vi "share data state machine.vi"(6 "Share data command":T7=enum."Write data", 8 "error in (no error)":errorcluster, 10 "Selected Shared Data":T3, 11 "Write data cluster in":T4) -> (0 "error out":errorcluster, 1 "Data from shared sources":T1 {"Sensor array"."scaled" format="%.2f"; "Sensor array"."voltage" format="%.4f"; "Time" format="%<%I:%M:%S%2u %p\n%m/%d/%Y>T"}, 2 "Available shared data":T5 {"Shared Data"."scaled" format="%.2f"}, 3 "My Data":T6 {"scaled" format="%.2f"}, 4 "Shared data names (unit)":string[](array[string]), 5 "read error":bool, 7 "Write data cluster out":T4)   [LabVIEW 2015]
uses:
  share data command.ctl
  shared data (name value unit).ctl
  write data cluster.ctl
  available share data.ctl
  selected shared data.ctl
  TCP DAQ/Sensor data.ctl
  DAQ configuration/sensor cluster.ctl
  Process Controller 3.0/Calibration and Function folders.ctl
  buffer.ctl
  <vilib>/Utility/config.llb/Read Key (Double).vi
  <vilib>/Utility/config.llb/Read Key (Path).vi
  <vilib>/Utility/config.llb/Read Key (U32).vi
  <vilib>/Utility/config.llb/Read Key (String).vi
  <vilib>/Utility/config.llb/Write Key (Double).vi
  <vilib>/Utility/config.llb/Write Key (Path).vi
  <vilib>/Utility/config.llb/Write Key (U32).vi
  <vilib>/Utility/config.llb/Write Key (String).vi
  <vilib>/Utility/config.llb/NI_LVConfig.lvlib
panel:
  out "my shared data file path":path
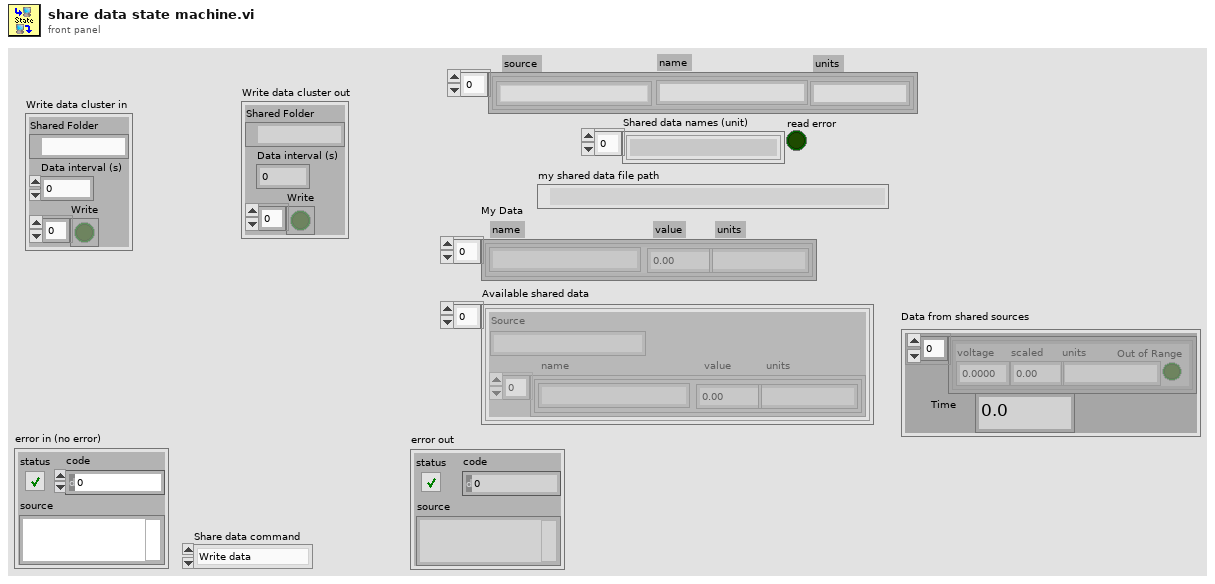
[diagram p1: front panel]
types:
  T1 = typedef "Sensor data.ctl" = cluster{" Sensor array":T2[], "Time":dbl}
  T2 = typedef "sensor cluster.ctl" = cluster{"voltage":sgl, "scaled":sgl, "units":string, "Out of Range":bool}
  T3 = typedef "selected shared data.ctl" = cluster{"Source":string, "name":string, "units":string}[]
  T4 = typedef "write data cluster.ctl" = cluster{"Data interval (s)":sgl, "Shared Folder":path, "Write":bool[]}
  T5 = typedef "available share data.ctl" = cluster{"Source":string, "Shared Data":T6}[]
  T6 = typedef "shared data (name value unit).ctl" = cluster{"name":string, "units":string, "scaled":sgl}[]
  T7 = typedef "share data command.ctl" = enum16{"Initialize from ini", "Update ini", "Write data", "Read data", "List my data", "List shared data", "Close"}
  T8 = typedef "Calibration and Function folders.ctl" = enum16{"Sensors", "Functions", "Config File", "PublicAppFolder", "New ini File", "Set Config File", "Delete ini File"}
  T9 = typedef "buffer.ctl" = enum16{"write", "read", "read merge"}
  T10 = cluster{"Controls[][0]":refnum<vi>, "Controls[][1]":refnum<vi>, "Controls[][2]":refnum<vi>}
  T11 = typedef "NI_LVConfig.lvlib/Config Data RefNum.ctl" = refnum<k1>
  T12 = cluster{"name":string, "units":string, "scaled":sgl}
  T13 = cluster{"name":string, cluster{"name":string, "units":string, "scaled":sgl}[]}
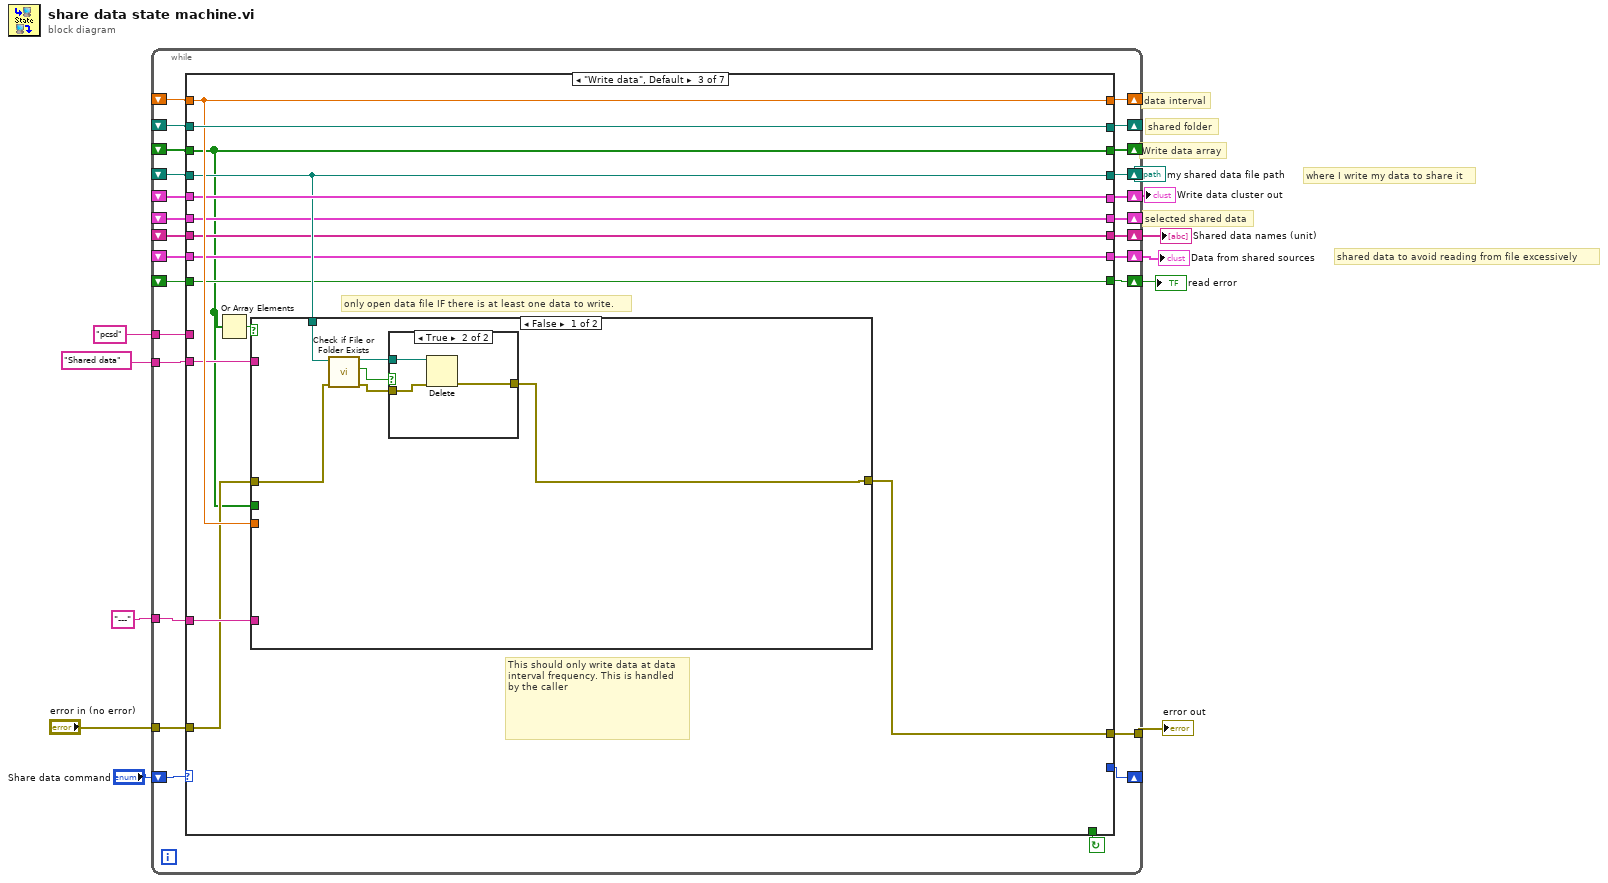
[diagram p0: block diagram]
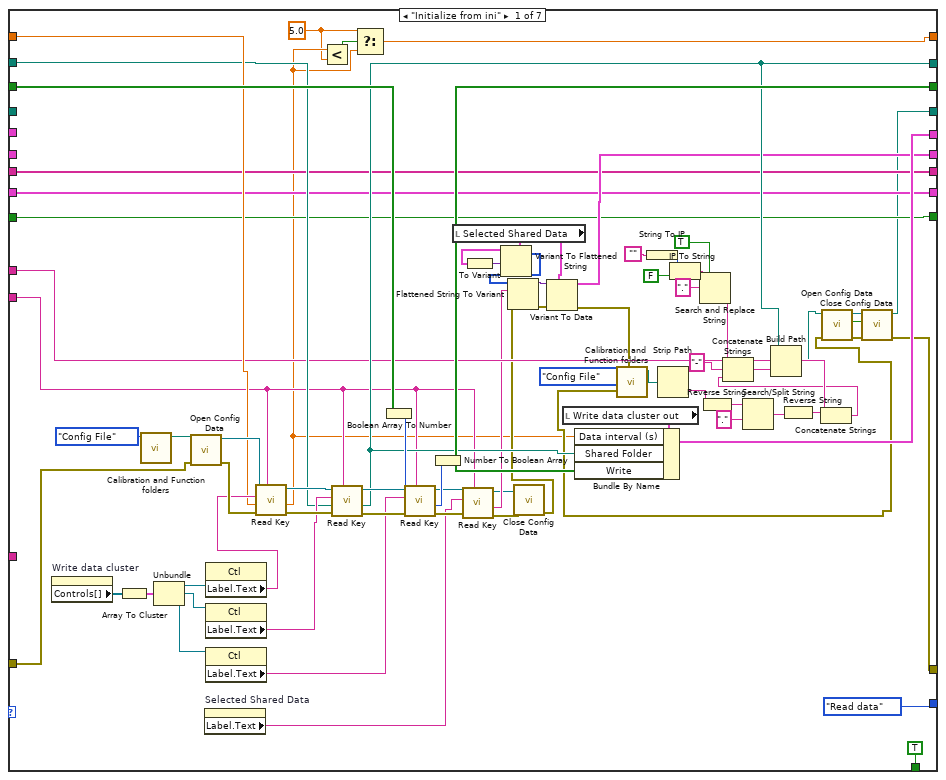
[diagram p2: hidden frame]
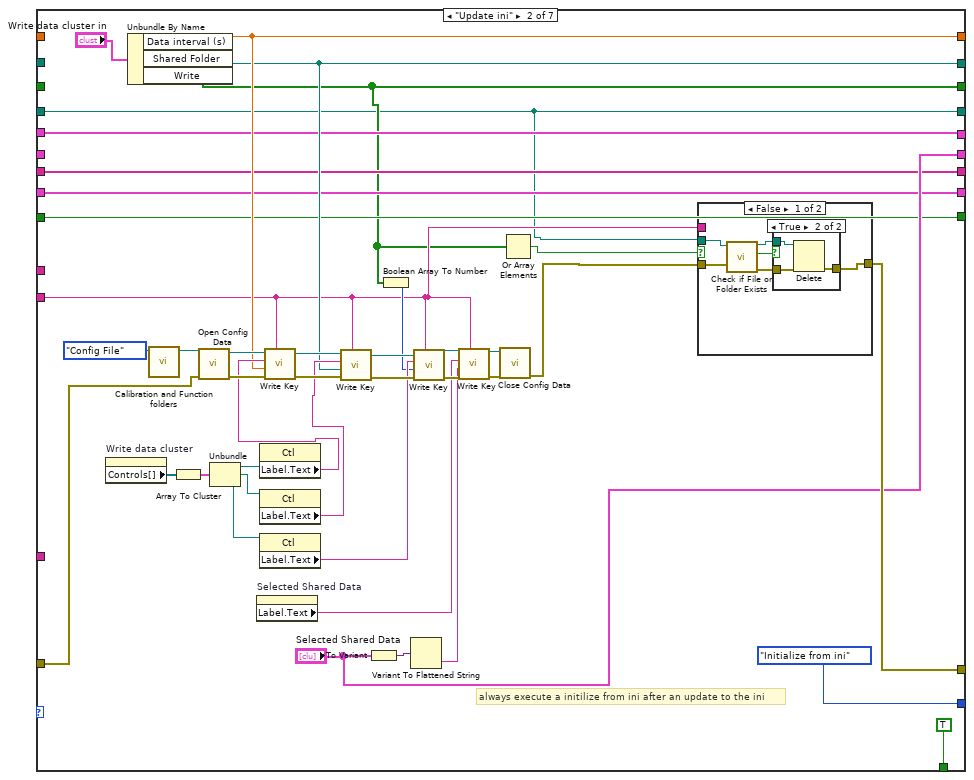
[diagram p3: hidden frame]
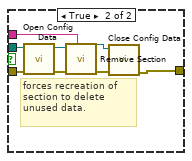
[diagram p5: hidden frame]
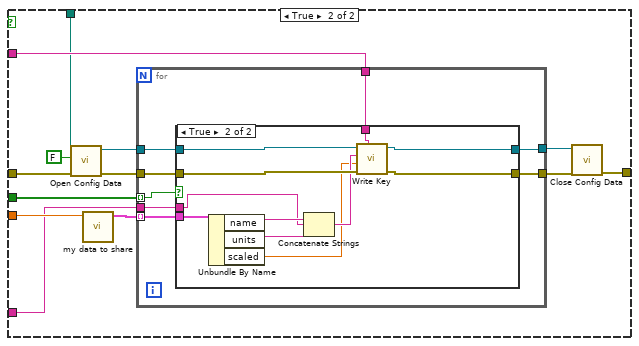
[diagram p7: hidden frame]
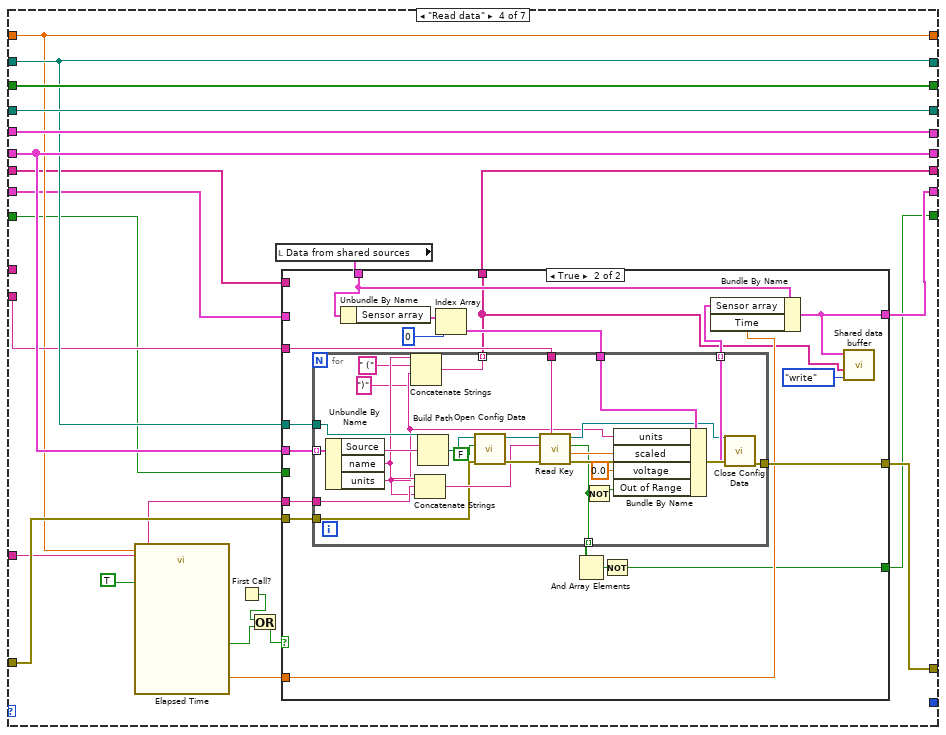
[diagram p9: hidden frame]
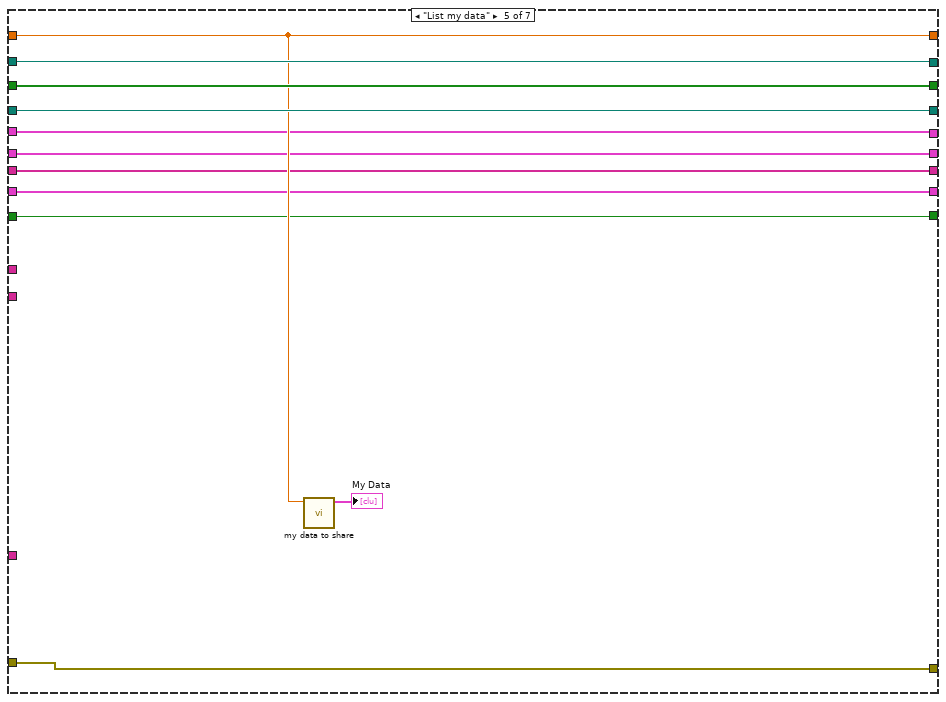
[diagram p11: hidden frame]
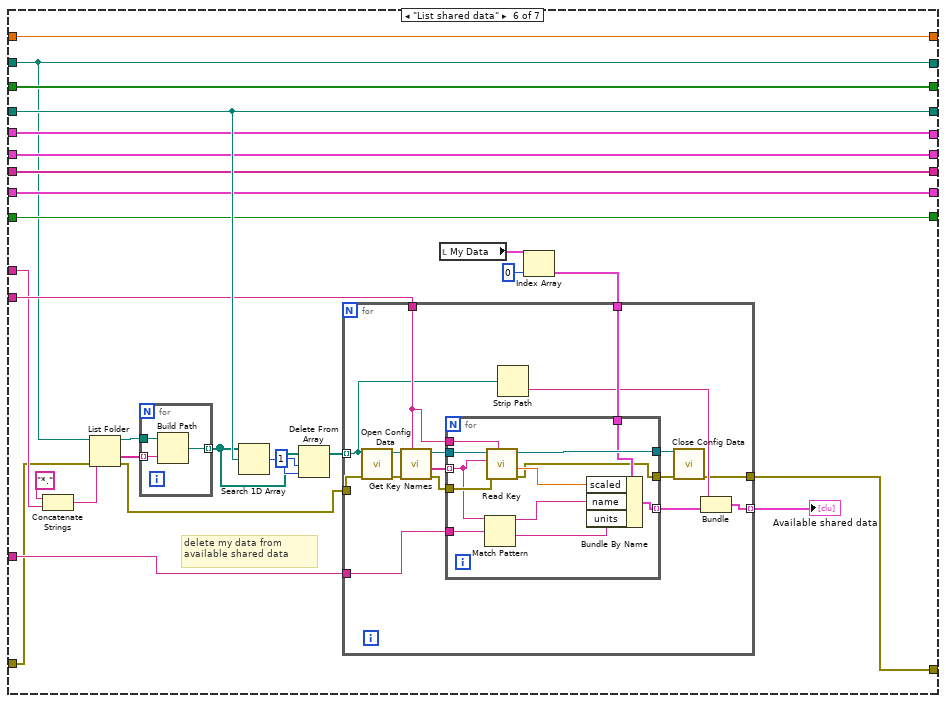
[diagram p12: hidden frame]
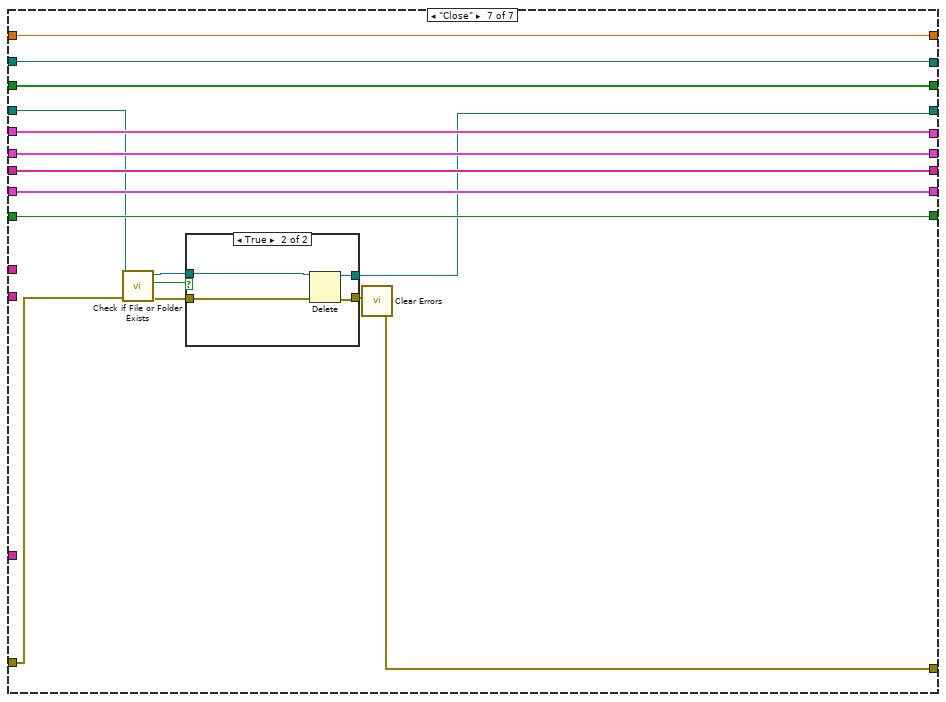
[diagram p13: hidden frame]
diagram:
  # "shared data to avoid reading from file excessively"
  # "selected shared data"
  # "Write data array"
  # "where I write my data to share it"
  # "shared folder"
  # "data interval"
  n1 = while {
    tunnel: [w37] -> w11
    tunnel: "error in (no error)" -> [w36]
    shift-right: [w35] -> _
    shift-left: _ -> [w34]
    shift-right: [w33] -> _
    shift-left: _ -> [w32]
    shift-right: [w31] -> w4
    shift-left: _ -> [w30]
    tunnel: "Shared data" ("section") -> [w29]
    shift-right: [w28] -> _
    shift-left: _ -> [w27]
    shift-right: [w26] -> w8
    shift-left: _ -> [w25]
    tunnel: "pcsd" ("pattern") -> [w24]
    shift-right: [w23] -> _
    shift-left: "Share data command" -> [w21]
    tunnel: "---" ("unit delimiter") -> [w20]
    shift-right: [w19] -> _
    shift-left: _ -> [w18]
    shift-right: [w17] -> w3
    shift-left: _ -> [w15]
    shift-right: [w16] -> w2
    shift-left: _ -> [w14]
    shift-right: [w13] -> w1
    shift-left: _ -> [w12]
    stop <- w22 continue-if-true
    n2 = case shown="\"Write data\", Default" w21 {
      tunnel: [w42 w128 w177 w243 w308 w324 w367] -> w37
      tunnel: w36 -> [w95 w144 w178 w244 w308 w309 w372]
      tunnel: [w40 w133 w183 w241 w303 w335 w382] -> w35
      tunnel: w34 -> [w81 _ w183 w241 w303 w335 w382]
      tunnel: [w79 w132 w184 w246 w307 w315 w381] -> w33
      tunnel: w32 -> [w80 _ w184 w246 w307 w315 w381]
      tunnel: [w44 w112 w179 w250 w306 w333 w368] -> w31
      tunnel: w30 -> [_ w112 w179 w250 w306 w333 w373]
      tunnel: w29 -> [w68 w126 w182 w245 _ w329 _]
      tunnel: [w83 w115 w172 w249 w305 w334 w380] -> w28
      tunnel: w27 -> [w87 _ w172 w249 w305 w334 w380]
      tunnel: [w78 w131 w181 w248 w302 w323 w379] -> w26
      tunnel: w25 -> [_ w131 w181 w248 w302 w323 w379]
      tunnel: w24 -> [w74 _ _ _ _ w321 _]
      tunnel: [share_data_command."Read data" ("Share data command") share_data_command."Initialize from ini" ("Share data command") _ _ _ _ _] -> w23
      tunnel: [TRUE TRUE _ _ _ _ _] -> w22
      tunnel: w20 -> [_ _ w180 w242 _ w320 _]
      tunnel: [w64 "Selected Shared Data" w176 w247 w301 w319 w377] -> w19
      tunnel: w18 -> [_ _ w176 w247 w301 w319 w377]
      tunnel: [w56 w119 w175 w239 w300 w318 w376] -> w17
      tunnel: [w55 w118 w174 w234 w299 w317 w375] -> w16
      tunnel: w15 -> [w56 w119 w175 w238 w300 w318 w376]
      tunnel: w14 -> [w55 w118 w174 w237 w299 w317 w375]
      tunnel: [w54 w117 w173 w233 w298 w316 w374] -> w13
      tunnel: w12 -> [w54 w117 w173 w232 w298 w316 w374]
      frame "Initialize from ini" {
        w38 = 5.0 ("t")
        n3 = property on="Write data cluster" class="Clust (strict)"() -> ("Controls[]"=w94:refnum<vi>[])  [unwired: 2 in, 2 out]
        n4 = Array To Cluster(array=w94) -> (cluster=w93:T10)
        n5 = call "Calibration and Function folders.vi"("Folder"=Calibration_and_Function_folders."Config File") -> ("Selected Folder"=w101:path)  [unwired: 9 in, 1 out]
        n6 = Unbundle(w93) -> ("Controls[][0]"=w92:refnum<vi>, "Controls[][1]"=w91:refnum<vi>, "Controls[][2]"=w90:refnum<vi>)
        n7 = call <vilib>:"Open Config Data.vi"("error in (no error)"=w95, "configuration file path"=w101) -> ("error out"=w102:errorcluster, "refnum"=w103:T11)  [unwired: 7 in, 1 out]
        n8 = property on="Selected Shared Data" class="Arr (strict)"() -> ("Label.Text"=w67:string)  [unwired: 2 in, 2 out]
        n9 = property class="Ctl"(reference=w92) -> ("Label.Text"=w89:string)  [unwired: 1 in, 2 out]
        n10 = property class="Ctl"(reference=w91) -> ("Label.Text"=w88:string)  [unwired: 1 in, 2 out]
        n11 = property class="Ctl"(reference=w90) -> ("Label.Text"=w85:string)  [unwired: 1 in, 2 out]
        n12 = call-poly <vilib>:"Read Key.vi"("section"=w68, "error in (no error)"=w102, "default value"=w81, "key"=w89, "refnum"=w103) -> ("error out"=w97:errorcluster, "value"=w39:dbl, "refnum out"=w99:T11)  [unwired: 3 in, 1 out]
        n13 = Less?(x=w39, y=w38) -> (x < y?=w41:bool)
        n14 = call-poly <vilib>:"Read Key.vi"("section"=w68, "error in (no error)"=w97, "default value"=w80, "key"=w88, "refnum"=w99) -> ("error out"=w96:errorcluster, "value"=w79:path, "refnum out"=w98:T11)  [unwired: 3 in, 1 out]
        n15 = Select(t=w38, s=w41, f=w39) -> (s? t:f=w40:dbl)
        n16 = Boolean Array To Number(Boolean array=w87) -> (number=w84:u32)
        n17 = call-poly <vilib>:"Read Key.vi"("section"=w68, "error in (no error)"=w96, "default value"=w84, "key"=w85, "refnum"=w98) -> ("error out"=w70:errorcluster, "value"=w86:u32, "refnum out"=w62:T11)  [unwired: 3 in, 1 out]
        n18 = Number To Boolean Array(number=w86) -> (Boolean array=w83:bool[])
        n19 = local read "Selected Shared Data"() -> (w57:T3)
        n20 = call-poly <vilib>:"Read Key.vi"("section"=w68, "error in (no error)"=w70, "key"=w67, "refnum"=w62) -> ("error out"=w69:errorcluster, "value"=w66:string, "refnum out"=w63:T11)  [unwired: 4 in, 1 out]
        n21 = To Variant(anything=w57) -> (Variant=w61:variant)
        n22 = Variant To Flattened String(Variant=w61) -> (1:w60:i16[])  [unwired: 1 out]
        n23 = call <vilib>:"Close Config Data.vi"("error in (no error)"=w69, "refnum"=w63) -> ("error out"=w59:errorcluster)  [unwired: 8 in, 1 out]
        n24 = Flattened String To Variant(4:w59, 6:w66, 7:w60) -> (0:w58:errorcluster, 3:w65:variant)
        n25 = Variant To Data(error in=w58, type=w57, Variant=w65) -> (data=w64:T3, error out=w43:errorcluster)
        n26 = local read "Write data cluster out"() -> (w82:T4)
        n27 = Bundle By Name(cluster=w82, "Data interval (s)"=w39, "Shared Folder"=w79, "Write"=w83) -> (w78:T4)
        n28 = call "Calibration and Function folders.vi"("Folder"=Calibration_and_Function_folders."Config File") -> ("Selected Folder"=w107:path)  [unwired: 9 in, 1 out]
        n29 = String To IP(1:"") -> (0:w111:u32)
        n30 = Strip Path(path=w107) -> (name=w75:string)  [unwired: 1 out]
        n31 = IP To String(1:FALSE ("dot notation? (F)"), 2:w111) -> (0:w105:string)
        n32 = Search and Replace String(replace all?=TRUE ("replace all? (F)"), input string=w105, search string=".") -> (result string=w51:string)  [unwired: 5 in, 3 out]
        n33 = Reverse String(1:w75) -> (0:w77:string)
        n34 = Search/Split String(string=w77, search string/char (-)=".") -> (match + rest of string=w71:string)  [unwired: 1 in, 2 out]
        n35 = Reverse String(1:w71) -> (0:w73:string)
        n36 = Concatenate Strings(w73, w74) -> (w72:string)
        n37 = Concatenate Strings(w51, "-" ("string"), w72) -> (w106:string)
        n38 = Build Path(base path=w79, name or relative path=w106) -> (appended path=w45:path)
        n39 = call <vilib>:"Open Config Data.vi"("error in (no error)"=w43, "configuration file path"=w45) -> ("error out"=w46:errorcluster, "file created?"=w47:bool, "refnum"=w48:T11)  [unwired: 7 in]
        n40 = call <vilib>:"Close Config Data.vi"("error in (no error)"=w46, "write file if changed (T)"=w47, "refnum"=w48) -> ("error out"=w42:errorcluster, "file path"=w44:path)  [unwired: 7 in]
      }
      frame "Update ini" {
        # "always execute a initilize from ini after an update to the ini"
        n41 = property on="Write data cluster" class="Clust (strict)"() -> ("Controls[]"=w142:refnum<vi>[])  [unwired: 2 in, 2 out]
        n42 = Unbundle By Name("Write data cluster in") -> ("Data interval (s)"=w133:sgl, "Shared Folder"=w132:path, "Write"=w115:bool[])
        n43 = call "Calibration and Function folders.vi"("Folder"=Calibration_and_Function_folders."Config File") -> ("Selected Folder"=w150:path)  [unwired: 9 in, 1 out]
        n44 = Array To Cluster(array=w142) -> (cluster=w141:T10)
        n45 = call <vilib>:"Open Config Data.vi"("error in (no error)"=w144, "configuration file path"=w150) -> ("error out"=w151:errorcluster, "refnum"=w152:T11)  [unwired: 7 in, 1 out]
        n46 = Unbundle(w141) -> ("Controls[][0]"=w140:refnum<vi>, "Controls[][1]"=w139:refnum<vi>, "Controls[][2]"=w138:refnum<vi>)
        n47 = property on="Selected Shared Data" class="Arr (strict)"() -> ("Label.Text"=w123:string)  [unwired: 2 in, 2 out]
        n48 = property class="Ctl"(reference=w140) -> ("Label.Text"=w137:string)  [unwired: 1 in, 2 out]
        n49 = property class="Ctl"(reference=w139) -> ("Label.Text"=w136:string)  [unwired: 1 in, 2 out]
        n50 = property class="Ctl"(reference=w138) -> ("Label.Text"=w135:string)  [unwired: 1 in, 2 out]
        n51 = call-poly <vilib>:"Write Key.vi"("section"=w126, "error in (no error)"=w151, "value"=w133, "key"=w137, "refnum"=w152) -> ("error out"=w146:errorcluster, "refnum out"=w148:T11)  [unwired: 4 in, 1 out]
        n52 = call-poly <vilib>:"Write Key.vi"("section"=w126, "error in (no error)"=w146, "value"=w132, "key"=w136, "refnum"=w148) -> ("error out"=w145:errorcluster, "refnum out"=w147:T11)  [unwired: 4 in, 1 out]
        n53 = To Variant(anything="Selected Shared Data") -> (Variant=w122:variant)
        n54 = Boolean Array To Number(Boolean array=w115) -> (number=w134:u32)
        n55 = Variant To Flattened String(Variant=w122) -> (data string=w121:string)  [unwired: 1 out]
        n56 = call-poly <vilib>:"Write Key.vi"("section"=w126, "error in (no error)"=w145, "value"=w134, "key"=w135, "refnum"=w147) -> ("error out"=w125:errorcluster, "refnum out"=w127:T11)  [unwired: 4 in, 1 out]
        n57 = call-poly <vilib>:"Write Key.vi"("section"=w126, "error in (no error)"=w125, "value"=w121, "key"=w123, "refnum"=w127) -> ("error out"=w124:errorcluster, "refnum out"=w114:T11)  [unwired: 4 in, 1 out]
        n58 = call <vilib>:"Close Config Data.vi"("error in (no error)"=w124, "refnum"=w114) -> ("error out"=w113:errorcluster)  [unwired: 8 in, 1 out]
        n59 = Or Array Elements(Boolean array=w115) -> (logical OR=w116:bool)
        n60 = case shown="False" w116 {
          tunnel: [w158 w168] -> w128
          tunnel: w112 -> [w157 w167]
          tunnel: w113 -> [w156 w166]
          tunnel: w126 -> [_ w163]
          frame False {
            n61 = call <vilib>:"Check if File or Folder Exists.vi"("error in (no error)"=w156, "path"=w157) -> ("error out"=w154:errorcluster, "file or folder exists?"=w155:bool, "dup path"=w153:path)  [unwired: 7 in]
            n62 = case shown="True" w155 {
              tunnel: [w159 w162] -> w158
              tunnel: w154 -> [w159 w161]
              tunnel: w153 -> [_ w160]
              frame False {
              }
              frame True {
                n63 = Delete(path (use dialog)=w160, error in=w161) -> (error out=w162:errorcluster)  [unwired: 3 in, 2 out]
              }
            }
          }
          frame True {
            # "forces recreation of section to delete unused data."
            n64 = call <vilib>:"Open Config Data.vi"("error in (no error)"=w166, "configuration file path"=w167) -> ("error out"=w164:errorcluster, "refnum"=w165:T11)  [unwired: 7 in, 1 out]
            n65 = call <vilib>:"Remove Section.vi"("section"=w163, "error in (no error)"=w164, "refnum"=w165) -> ("error out"=w169:errorcluster, "refnum out"=w170:T11)  [unwired: 6 in, 1 out]
            n66 = call <vilib>:"Close Config Data.vi"("error in (no error)"=w169, "refnum"=w170) -> ("error out"=w168:errorcluster)  [unwired: 8 in, 1 out]
          }
        }
      }
      frame "Write data", Default {
        # "only open data file IF there is at least one data to write."
        # "This should only write data at data interval frequency. This is handled by the caller"
        n67 = Or Array Elements(Boolean array=w172) -> (logical OR=w171:bool)
        n68 = case shown="False" w171 {
          tunnel: w183 -> [_ w207]
          tunnel: w182 -> [_ w205]
          tunnel: w172 -> [_ w204]
          tunnel: w180 -> [_ w203]
          tunnel: w179 -> [w190 w202]
          tunnel: w178 -> [w185 w201]
          tunnel: [w186 w196] -> w177
          frame False {
            n69 = call <vilib>:"Check if File or Folder Exists.vi"("error in (no error)"=w185, "path"=w190) -> ("error out"=w187:errorcluster, "file or folder exists?"=w189:bool, "dup path"=w188:path)  [unwired: 7 in]
            n70 = case shown="True" w189 {
              tunnel: w188 -> [_ w194]
              tunnel: w187 -> [w191 w193]
              tunnel: [w191 w192] -> w186
              frame False {
              }
              frame True {
                n71 = Delete(path (use dialog)=w194, error in=w193) -> (error out=w192:errorcluster)  [unwired: 3 in, 2 out]
              }
            }
          }
          frame True {
            n72 = call <vilib>:"Open Config Data.vi"("error in (no error)"=w201, "create file if necessary (T)"=FALSE, "configuration file path"=w202) -> ("error out"=w200:errorcluster, "refnum"=w199:T11)  [unwired: 6 in, 1 out]
            n73 = call "my data to share.vi"("Data interval (s)"=w207) -> ("Shared Data"=w206:T6)  [unwired: 10 in]
            n74 = for {
              tunnel: [w215] -> w198
              tunnel: w199 -> [w214]
              tunnel: w200 -> [w213]
              tunnel: [w212] -> w197
              tunnel: w206 -> [w209] mode=indexing
              tunnel: w205 -> [w211]
              tunnel: w204 -> [w210] mode=indexing
              tunnel: w203 -> [w208]
              n75 = case shown="True" w210 {
                tunnel: [w217 w228] -> w215
                tunnel: w214 -> [w217 w227]
                tunnel: w213 -> [w216 w226]
                tunnel: [w216 w225] -> w212
                tunnel: w211 -> [_ w224]
                tunnel: w209 -> [_ w223]
                tunnel: w208 -> [_ w218]
                frame False {
                }
                frame True {
                  n76 = Unbundle By Name(w223) -> ("name"=w222:string, "units"=w221:string, "scaled"=w219:sgl)
                  n77 = Concatenate Strings(w222, w218, w221) -> (w220:string)
                  n78 = call-poly <vilib>:"Write Key.vi"("section"=w224, "error in (no error)"=w226, "value"=w219, "key"=w220, "refnum"=w227) -> ("error out"=w225:errorcluster, "refnum out"=w228:T11)  [unwired: 4 in, 1 out]
                }
              }
            }
            n79 = call <vilib>:"Close Config Data.vi"("error in (no error)"=w197, "refnum"=w198) -> ("error out"=w196:errorcluster)  [unwired: 8 in, 1 out]
          }
        }
      }
      frame "Read data" {
        n80 = call "Elapsed Time"("Time Target (s)"=w241, "Auto Reset"=TRUE ("Reset")) -> ("Present (s)"=w236:dbl, "Time has Elapsed"=w230:bool)  [unwired: 10 in, 6 out]
        n81 = First Call?() -> (First Call?: T/F=w231:bool)
        n82 = Or(x=w231, y=w230) -> (x .or. y?=w229:bool)
        n83 = local read "Data from shared sources"() -> (w235:T1)
        n84 = case shown="True" w229 {
          tunnel: w247 -> [_ w272]
          tunnel: w246 -> [_ w271]
          tunnel: w245 -> [_ w270]
          tunnel: w244 -> [w254 w269]
          tunnel: [w254 w268] -> w243
          tunnel: w242 -> [_ w267]
          tunnel: [w253 w255] -> w239
          tunnel: w238 -> [w253 _]
          tunnel: w237 -> [w252 _]
          tunnel: w236 -> [_ w261]
          tunnel: w235 -> [_ w262]
          tunnel: [w252 w260] -> w234
          tunnel: [w251 w256] -> w233
          tunnel: w232 -> [w251 _]
          frame False {
          }
          frame True {
            n85 = Unbundle By Name(w262) -> ("Sensor array"=w266:T2[])
            n86 = Index Array(array=w266, index=0) -> (element=w264:T2)
            n87 = for {
              tunnel: w272 -> [w297] mode=indexing
              tunnel: w271 -> [w285]
              tunnel: w270 -> [w294]
              tunnel: w269 -> [w286]
              tunnel: [w291] -> w268
              tunnel: w264 -> [w290]
              tunnel: w267 -> [w289]
              tunnel: [w284] -> w263 mode=indexing
              tunnel: [w277] -> w255 mode=indexing
              tunnel: [w274] -> w258 mode=indexing
              n88 = Unbundle By Name(w297) -> ("Source"=w296:string, "name"=w281:string, "units"=w279:string)
              n89 = Concatenate Strings(w281, " (" ("string"), w279, ")" ("string")) -> (w277:string)
              n90 = Concatenate Strings(w281, w289, w279) -> (w288:string)
              n91 = Build Path(base path=w285, name or relative path=w296) -> (appended path=w295:path)
              n92 = call <vilib>:"Open Config Data.vi"("error in (no error)"=w286, "create file if necessary (T)"=FALSE, "configuration file path"=w295) -> ("error out"=w293:errorcluster, "refnum"=w283:T11)  [unwired: 6 in, 1 out]
              n93 = call-poly <vilib>:"Read Key.vi"("section"=w294, "error in (no error)"=w293, "key"=w288, "refnum"=w283) -> ("error out"=w292:errorcluster, "value"=w287:dbl, "found?"=w274:bool, "refnum out"=w282:T11)  [unwired: 4 in]
              n94 = Not(x=w274) -> (.not. x?=w273:bool)
              n95 = Bundle By Name(cluster=w290, "units"=w279, "scaled"=w287, "voltage"=sgl 0.0, "Out of Range"=w273) -> (w284:T2)
              n96 = call <vilib>:"Close Config Data.vi"("error in (no error)"=w292, "refnum"=w282) -> ("error out"=w291:errorcluster)  [unwired: 8 in, 1 out]
            }
            n97 = And Array Elements(Boolean array=w258) -> (logical AND=w257:bool)
            n98 = Not(x=w257) -> (.not. x?=w256:bool)
            n99 = Bundle By Name(cluster=w262, "Sensor array"=w263, "Time"=w261) -> (w260:T1)
            n100 = call "Shared data buffer.vi"("command"=buffer."write", "Shared data names (unit) in"=w255, "Data from shared sources in"=w260) -> ()  [unwired: 6 in, 3 out]
          }
        }
      }
      frame "List my data" {
        n101 = call "my data to share.vi"("Data interval (s)"=w303) -> ("Shared Data"=→"My Data":T6)  [unwired: 10 in]
      }
      frame "List shared data" {
        # "delete my data from available shared data"
        n102 = Concatenate Strings("*." ("pattern"), w321) -> (w314:string)
        n103 = List Folder(path=w315, pattern=w314, error in=w309) -> (path out=w313:path, filenames=w312:string[], error out=w310:errorcluster)  [unwired: 1 in, 1 out]
        n104 = for {
          tunnel: w313 -> [w338]
          tunnel: w312 -> [w337] mode=indexing
          tunnel: [w336] -> w311 mode=indexing
          n105 = Build Path(base path=w338, name or relative path=w337) -> (appended path=w336:path)
        }
        n106 = Search 1D Array(1D array=w311, element=w333) -> (index of element=w332:i32)  [unwired: 1 in]
        n107 = Delete From Array(array=w311, length=1, index=w332) -> (array with subset deleted=w330:path[])  [unwired: 1 out]
        n108 = local read "My Data"() -> (w328:T6)
        n109 = Index Array(array=w328, index=0) -> (element=w326:T12)
        n110 = for {
          tunnel: w330 -> [w345] mode=indexing
          tunnel: w329 -> [w351]
          tunnel: w326 -> [w347]
          tunnel: [w343] -> w325 mode=indexing
          tunnel: w310 -> [w342]
          tunnel: [w340] -> w324
          tunnel: w320 -> [w339]
          n111 = call <vilib>:"Open Config Data.vi"("error in (no error)"=w342, "configuration file path"=w345) -> ("error out"=w354:errorcluster, "refnum"=w353:T11)  [unwired: 7 in, 1 out]
          n112 = call <vilib>:"Get Key Names.vi"("section"=w351, "error in (no error)"=w354, "refnum"=w353) -> ("error out"=w349:errorcluster, "key names"=w350:string[], "refnum out"=w352:T11)  [unwired: 5 in, 1 out]
          n113 = for {
            tunnel: w352 -> [w366]
            tunnel: w351 -> [w365]
            tunnel: w350 -> [w358] mode=indexing
            tunnel: w349 -> [w364]
            tunnel: [w363] -> w348
            tunnel: w347 -> [w362]
            tunnel: [w360] -> w346 mode=indexing
            tunnel: [w359] -> w341
            tunnel: w339 -> [w355]
            n114 = Match Pattern(string=w358, regular expression=w355) -> (before substring=w357:string, after substring=w356:string)  [unwired: 1 in, 2 out]
            n115 = call-poly <vilib>:"Read Key.vi"("section"=w365, "error in (no error)"=w364, "key"=w358, "refnum"=w366) -> ("error out"=w359:errorcluster, "value"=w361:dbl, "refnum out"=w363:T11)  [unwired: 4 in, 1 out]
            n116 = Bundle By Name(cluster=w362, "scaled"=w361, "name"=w357, "units"=w356) -> (w360:T12)
          }
          n117 = Strip Path(path=w345) -> (name=w344:string)  [unwired: 1 out]
          n118 = call <vilib>:"Close Config Data.vi"("error in (no error)"=w341, "refnum"=w348) -> ("error out"=w340:errorcluster)  [unwired: 8 in, 1 out]
          n119 = Bundle("name"=w344, w346) -> (w343:T13)  [unwired: 1 in]
        }
        "Available shared data" <- w325
      }
      frame "Close" {
        n120 = call <vilib>:"Check if File or Folder Exists.vi"("error in (no error)"=w372, "path"=w373) -> ("error out"=w369:errorcluster, "file or folder exists?"=w371:bool, "dup path"=w370:path)  [unwired: 7 in]
        n121 = case shown="True" w371 {
          tunnel: [w384 w388] -> w378
          tunnel: w370 -> [w383 w387]
          tunnel: w369 -> [w384 w386]
          tunnel: [w383 w385] -> w368
          frame False {
          }
          frame True {
            n122 = Delete(path (use dialog)=w387, error in=w386) -> (deleted path=w385:path, error out=w388:errorcluster)  [unwired: 3 in, 1 out]
          }
        }
        n123 = call <vilib>:"Clear Errors.vi"("error in (no error)"=w378) -> ("error out"=w367:errorcluster)  [unwired: 5 in, 1 out]
      }
    }
  }
  "error out" <- w11
  "my shared data file path" <- w4
  "Write data cluster out" <- w8
  "Shared data names (unit)" <- w3
  "Data from shared sources" <- w2
  "read error" <- w1
